vi "ignitePilot.vi"(8 "error in":errorcluster, 9 "Boiler Simulation Controls":refnum<vi>, 10 "Boiler Controls":refnum<vi>, 11 "Boiler Status Indicators":refnum<vi>) -> (0 "error out":errorcluster, 3 "pilotOn?":bool)   [LabVIEW 2024]
uses:
  Controls/Boiler Simulation Controls.ctl
  Controls/Boiler Status Indicators.ctl
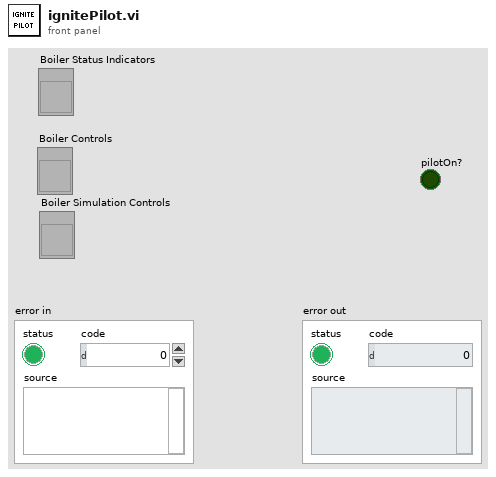
[diagram p1: front panel]
types:
  T1 = typedef "Boiler Controls.ctl" = cluster{"Boiler Reset":bool, "Start Sequence":bool, "Pilot":bool, "Shutdown":bool, "Fuel Valve Position":dbl}
  T2 = typedef "Boiler Status Indicators.ctl" = cluster{"Status":string, "Primary Fan":bool, "Natural Gas Valve":bool, "Pilot":bool, "Fuel Valve":bool, "Forced Draft Fan":bool, "Time Count":dbl}
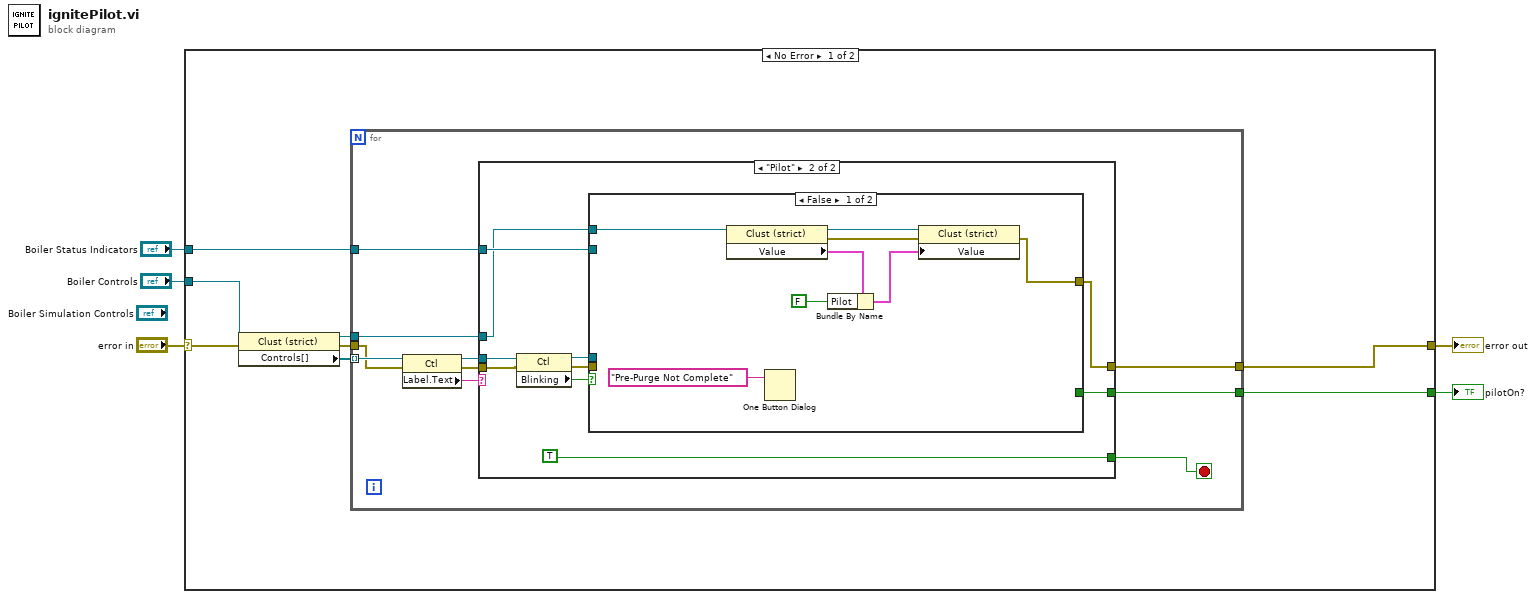
[diagram p0: block diagram]
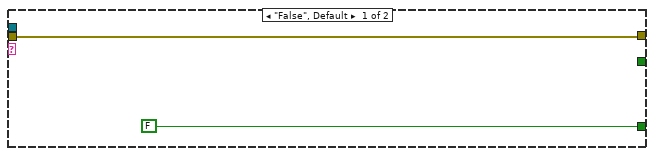
[diagram p2: hidden frame]
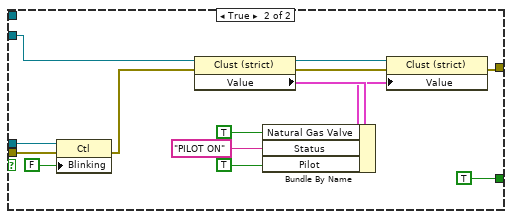
[diagram p3: hidden frame]
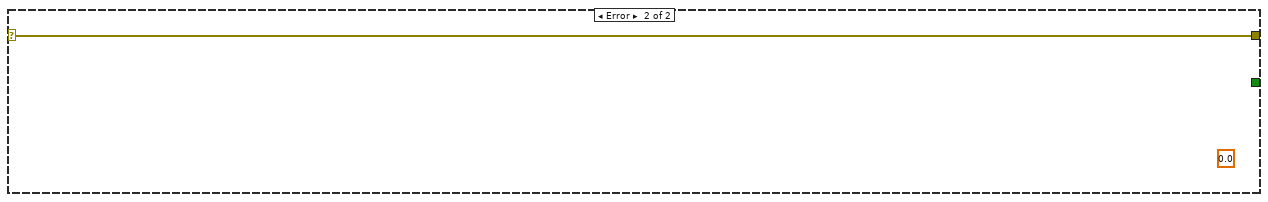
[diagram p4: hidden frame]
diagram:
  n1 = case shown="No Error" "error in" {
    selector: "error in" -> [w9 w58]
    tunnel: [w11 w58] -> w4
    tunnel: "Boiler Status Indicators" -> [w8 _]
    tunnel: "Boiler Controls" -> [w10 _]
    tunnel: [w7 _] -> w1
    frame No Error {
      n2 = property class="Clust (strict)"(reference=w10, error in=w9) -> (reference out=w6:refnum<vi>, error out=w12:errorcluster, "Controls[]"=w13:refnum<vi>[])
      n3 = for {
        tunnel: w13 -> [w23] mode=indexing
        tunnel: w12 -> [w21]
        tunnel: [w18] -> w11
        tunnel: w8 -> [w16]
        tunnel: [w15] -> w7
        tunnel: w6 -> [w14]
        stop <- w17 stop-if-true
        n4 = property class="Ctl"(reference=w23, error in=w21) -> (reference out=w20:refnum<vi>, error out=w19:errorcluster, "Label.Text"=w22:string)
        n5 = case shown="\"Pilot\"" w22 {
          tunnel: w20 -> [_ w35]
          tunnel: w19 -> [w25 w34]
          tunnel: [w25 w29] -> w18
          tunnel: [FALSE TRUE] -> w17
          tunnel: w16 -> [_ w30]
          tunnel: [_ w27] -> w15
          tunnel: w14 -> [_ w26]
          frame "False", Default {
          }
          frame "Pilot" {
            n6 = property class="Ctl"(reference=w35, error in=w34) -> (reference out=w28:refnum<vi>, error out=w31:errorcluster, "Blinking"=w32:bool)
            n7 = case shown="False" w32 {
              tunnel: w31 -> [_ w46]
              tunnel: w30 -> [_ w51]
              tunnel: [w36 w49] -> w29
              tunnel: w28 -> [_ w48]
              tunnel: [_ TRUE] -> w27
              tunnel: w26 -> [w38 _]
              frame False {
                n8 = property class="Clust (strict)"(reference=w38) -> (reference out=w42:refnum<vi>, error out=w41:errorcluster, "Value"=w40:T1)  [unwired: 1 in]
                n9 = One Button Dialog(message="Pre-Purge Not Complete") -> ()  [unwired: 1 in, 1 out]
                n10 = Bundle By Name(cluster=w40, "Pilot"=FALSE) -> (w39:T1)
                n11 = property class="Clust (strict)"(reference=w42, error in=w41, "Value"=w39) -> (error out=w36:errorcluster)  [unwired: 1 out]
              }
              frame True {
                n12 = property class="Ctl"(reference=w48, error in=w46, "Blinking"=FALSE) -> (error out=w45:errorcluster)  [unwired: 1 out]
                n13 = property class="Clust (strict)"(reference=w51, error in=w45) -> (reference out=w57:refnum<vi>, error out=w56:errorcluster, "Value"=w55:T2)
                n14 = Bundle By Name(cluster=w55, "Natural Gas Valve"=TRUE ("Primary Fan"), "Status"="PILOT ON", "Pilot"=TRUE) -> (w54:T2)
                n15 = property class="Clust (strict)"(reference=w57, error in=w56, "Value"=w54) -> (error out=w49:errorcluster)  [unwired: 1 out]
              }
            }
          }
        }
      }
    }
    frame Error {
      (unwired) 0.0
    }
  }
  "error out" <- w4
  "pilotOn?" <- w1
